vi "CONV String to 2D Hexidecimal.vi"(0 "String":string, 1 "Delimiters (,;)":string=",;") -> (6 "2-D Hexidecimal":u32[][](array[numeric]) format="%.0x")   [LabVIEW 2017]
doc: "This routine converts a string list to a 2-D U32 Hexidecimal Array. There should be exactly 2 characters in the Delimiters field. The first is the Column delimiter, and the Second is the Row delimiter.\n\nExample:\n\nString: 1,2,3;4,5,6\nDelimiters: ,;\n\nOutput\n\n1 2 3\n4 5 6"
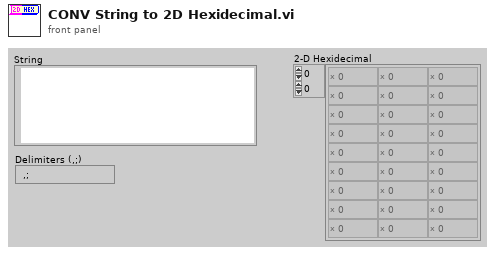
[diagram p1: front panel]
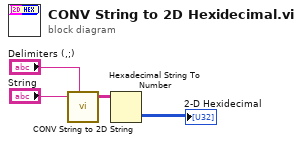
[diagram p0: block diagram]
diagram:
  n1 = call "CONV String to 2D String.vi"("String"="String", "Delimiters (,;)"="Delimiters (,;)") -> ("2-D String"=w2:string[][])  [unwired: 7 in]
  n2 = Hexadecimal String To Number(string=w2) -> (number=→"2-D Hexidecimal":u32[][])  [unwired: 2 in, 1 out]
